vi "API - Stream - Download One Datapoint from One ADC Channel.vi"(8 "error in":errorcluster, 11 "DAQiFi Device Properties In":T1) -> (0 "error out":errorcluster, 2 "Analog Voltage (V)":dbl, 3 "DAQiFi Device Properties Out":T1)   [LabVIEW 2021]
doc: "Download a single data point from one ADC channel."
uses:
  TypeDefs/TypeDef - Cluster of DAQiFi Device Properties.ctl
  TypeDefs/Enum - Connection Type.ctl
  TCP - Asynchronous Read of One JSON Message.vi
  USB - Asynchronous Read of One JSON Message.vi
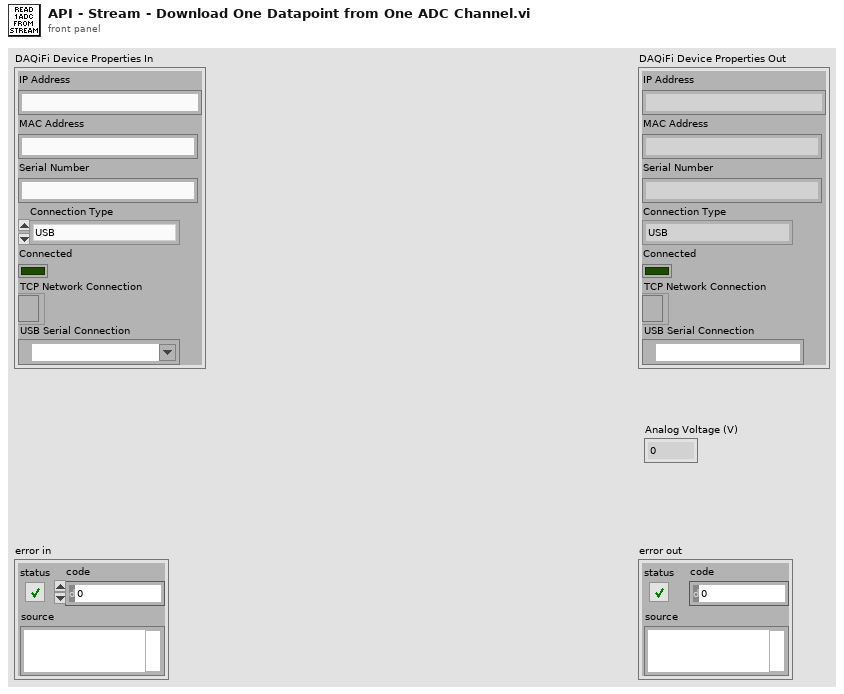
[diagram p1: front panel]
types:
  T1 = typedef "TypeDef - Cluster of DAQiFi Device Properties.ctl" = cluster{"IP Address":string, "MAC Address":string, "Serial Number":string, "Connection Type":T2, "Connected":bool, "TCP Network Connection":refnum<k5>, "USB Serial Connection":refnum<visa-resource-name>}
  T2 = typedef "Enum - Connection Type.ctl" = enum16{"USB", "TCP"}
  T3 = typedef "TypeDef - Cluster Representing Decoded JSON Message.ctl" = cluster{"timestamp":u64, "adc":cluster{"time":i32, "ch":i32, "data":i32}[], "dio":cluster{"time":i32, "mask":i32, "data":u16}[]}
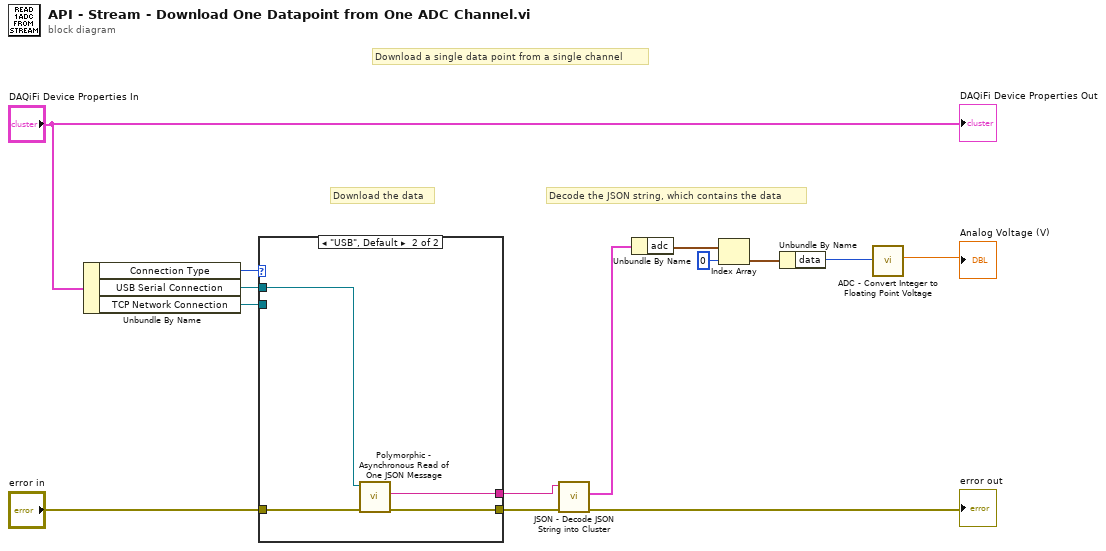
[diagram p0: block diagram]
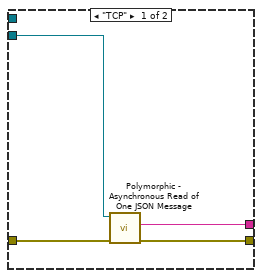
[diagram p2: hidden frame]
diagram:
  # "Download the data"
  # "Download a single data point from a single channel"
  # "Decode the JSON string, which contains the data"
  n1 = Unbundle By Name("DAQiFi Device Properties In") -> ("Connection Type"=w4:T2, "USB Serial Connection"=w1:refnum<visa-resource-name>, "TCP Network Connection"=w3:refnum<k5>)
  n2 = case shown="\"USB\", Default" w4 {
    tunnel: "error in" -> [w18 w22]
    tunnel: [w17 w21] -> w6
    tunnel: w3 -> [w16 _]
    tunnel: [w15 w20] -> w2
    tunnel: w1 -> [_ w19]
    frame "TCP" {
      n3 = call-poly "Polymorphic - Asynchronous Read of One JSON Message.vi"("error in"=w18, "TCP Network Connection in"=w16) -> ("error out"=w17:errorcluster, "Received JSON Message"=w15:string)  [unwired: 7 in, 1 out]
    }
    frame "USB", Default {
      n4 = call-poly "Polymorphic - Asynchronous Read of One JSON Message.vi"("error in"=w22, "VISA resource name in"=w19) -> ("error out"=w21:errorcluster, "Received JSON Message"=w20:string)  [unwired: 7 in, 1 out]
    }
  }
  n5 = call "JSON - Decode JSON String into Cluster.vi"("error in"=w6, "JSON String"=w2) -> ("error out"=→"error out":errorcluster, "Data out"=w9:T3)  [unwired: 8 in]
  n6 = Unbundle By Name(w9) -> ("adc"=w10:cluster{"time":i32, "ch":i32, "data":i32}[])
  n7 = Index Array(array=w10, index=0) -> (element=w12:cluster{"time":i32, "ch":i32, "data":i32})
  n8 = Unbundle By Name(w12) -> ("data"=w13:i32)
  n9 = call "ADC - Convert Integer to Floating Point Voltage.vi"("Analog Integer Value In"=w13) -> ("Analog Voltage (V)"=→"Analog Voltage (V)":dbl)  [unwired: 10 in]
  "DAQiFi Device Properties Out" <- "DAQiFi Device Properties In"
